vi "UDT_application_ClustertoRawString.vi"() -> (3 "Unit Test Framework Results":T1)   [LabVIEW 2017]
doc: "Use this template to create a user-defined test VI. Define your test requirements and wire the results to the <b>Result (Test)</b> control. Do not modify the <b>Unit Test Framework Results</b> indicator."
uses:
  <vilib>/utf/common/utf_test_result_troll.ctl
  <vilib>/utf/common/utf_test_result.ctl
  <vilib>/utf/common/utf_test_result_failure.ctl
  <vilib>/utf/common/utf_test_comparison_operators.ctl
  <vilib>/utf/common/utf_vi_tag.ctl
  RT/TypeDefs/dataOut.ctl
  <vilib>/Control Software Solutions Ltd/UTF Helper/SubVIs/UTF String Equals.vi
  <vilib>/Control Software Solutions Ltd/UTF Helper/Unit Test Helper.lvlib
  <vilib>/utf/NI_UnitTestFramework.lvlib
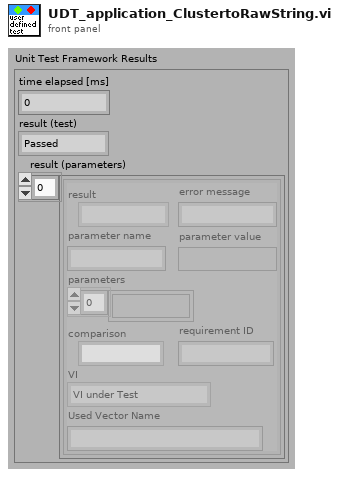
[diagram p1: front panel]
types:
  T1 = typedef "NI_UnitTestFramework.lvlib/utf_test_result_troll.ctl" = cluster{"time elapsed [ms]":u32, "result (test)":T2, "result (parameters)":T3[]}
  T2 = typedef "NI_UnitTestFramework.lvlib/utf_test_result.ctl" = enum16{"Passed", "Failed", "Error", "Skipped", "Not Processed"}
  T3 = typedef "NI_UnitTestFramework.lvlib/utf_test_result_failure.ctl" = cluster{"result":T2, "error message":string, "parameter name":string, "parameter value":variant, "parameters":variant[], "comparison":T4, "requirement ID":string, "VI":T5, "Used Vector Name":string}
  T4 = typedef "NI_UnitTestFramework.lvlib/utf_test_comparison_operators.ctl" = enum16{"=", "!=", ">", ">=", "<", "<=", "range", "symmetric tolerance", "asymmetric tolerance", "string contains", "string not contain", "array size", "string length", "array range", "by element", "array range (limit array)", "user-defined", "array contains", "array not contain", "vector length", "= (elm)", "!= (elm)", "= (case insensitive)", "!= (case insensitive)"}
  T5 = typedef "NI_UnitTestFramework.lvlib/utf_vi_tag.ctl" = enum16{"Setup VI", "VI under Test", "Teardown VI"}
  T6 = typedef "dataOut.ctl" = cluster{"X0pos":dbl, "Y0pos":dbl, "Z0pos":dbl, "Fx":dbl, "Fy":dbl, "Fz":dbl, "Encoder1":i32, "Encoder2":i32, "Pot1":dbl, "Pot2":dbl, "Theta0":dbl, "Theta1":dbl, "X1pos":dbl, "Y1pos":dbl, "Z1pos":dbl, "X2pos":dbl, "Y2pos":dbl, "Z2pos":dbl, "ErrorOccurred":bool}
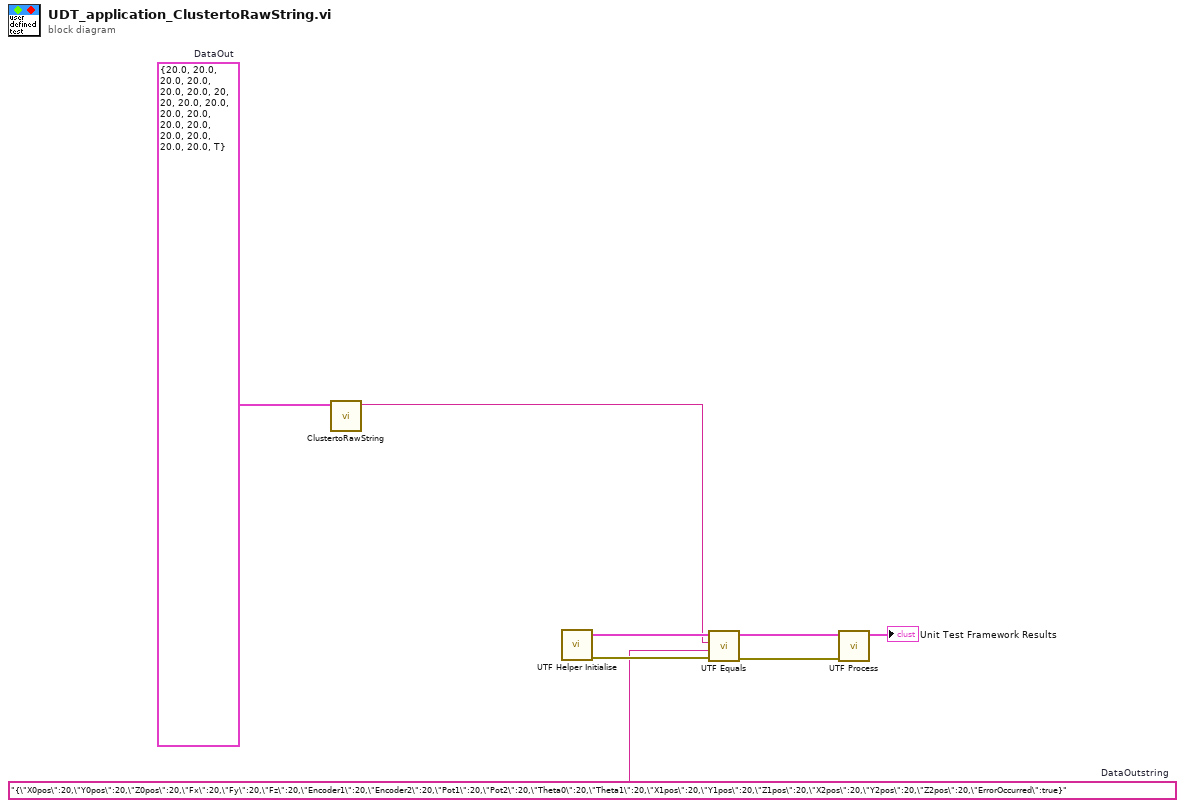
[diagram p0: block diagram]
diagram:
  w1 = "{\"X0pos\":20,\"Y0pos\":20,\"Z0pos\":20,\"Fx\":20,\"Fy\":20,\"Fz\":20,\"Encoder1\":20,\"Encoder2\":20,\"Pot1\":20,\"Pot2\":20,\"Theta0\":20,\"Theta1\":20,\"X1pos\":20,\"Y1pos\":20,\"Z1pos\":20,\"X2pos\":20,\"Y2pos\":20,\"Z2pos\":20,\"ErrorOccurred\":true}"  # DataOutstring
  w8 = T6 {"X0pos"=20.0, "Y0pos"=20.0, "Z0pos"=20.0, "Fx"=20.0, "Fy"=20.0, "Fz"=20.0, "Encoder1"=20, "Encoder2"=20, "Pot1"=20.0, "Pot2"=20.0, "Theta0"=20.0, "Theta1"=20.0, "X1pos"=20.0, "Y1pos"=20.0, "Z1pos"=20.0, "X2pos"=20.0, "Y2pos"=20.0, "Z2pos"=20.0, "ErrorOccurred"=TRUE}  # DataOut
  n1 = call "ClustertoRawString.vi"("DataOut"=w8) -> ("DataOutstring"=w2:string)  [unwired: 9 in, 1 out]
  n2 = call <vilib>:"UTF Helper Initialise.vi"() -> ("error out"=w3:errorcluster, "results array"=w4:T3[])  [unwired: 10 in]
  n3 = call-poly <vilib>:"UTF Equals.vi"("error in (no error)"=w3, "Test Value"=w1, "Input"=w2, "Input Results"=w4) -> ("error out"=w5:errorcluster, "Output Results"=w6:T3[])  [unwired: 6 in]
  n4 = call <vilib>:"UTF Process.vi"("error in (no error)"=w5, "results array"=w6) -> ("Unit Test Framework Results"=→"Unit Test Framework Results":T1)  [unwired: 9 in]
